vi "Globals.vi"() -> ()   [LabVIEW 2018]
panel:
  out "Slide":dbl
  out "input":string[][](array[string])
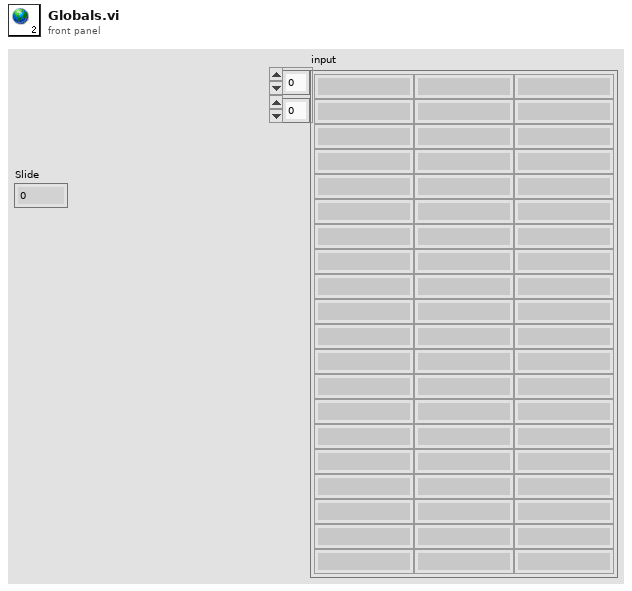
[diagram p1: front panel]
diagram:
